vi "ev GoTo.vi"(8 "error in (no error)":errorcluster, 11 "LF2R IDE in":refnum<class "Main Panel.lvclass">) -> (0 "error out":errorcluster, 3 "LF2R IDE out":refnum<class "Main Panel.lvclass">)   [LabVIEW 2018, in "Main Panel.lvlib" / "Main Panel.lvclass"]
uses:
  Main Panel.lvclass
  Main Panel.lvclass/Main Panel.ctl
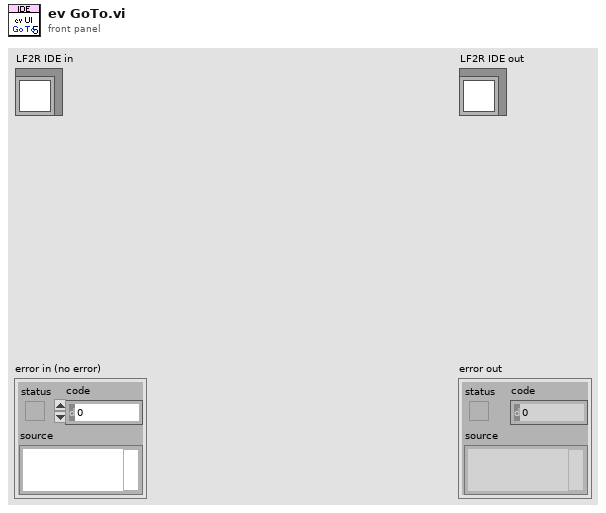
[diagram p1: front panel]
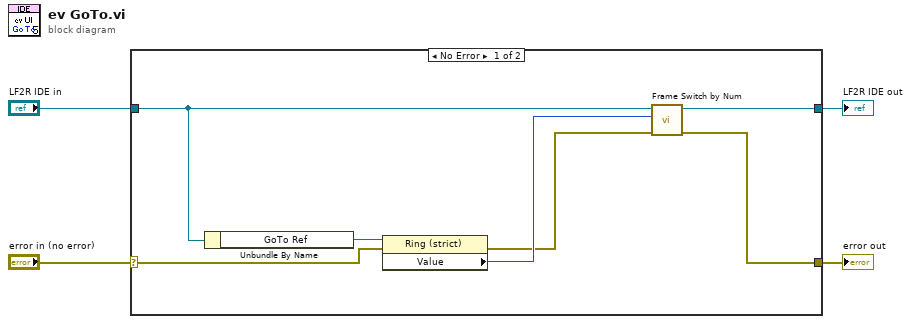
[diagram p0: block diagram]
diagram:
  n1 = case shown="No Error" "error in (no error)" {
    selector: "error in (no error)" -> [w7 w13]
    tunnel: [w5 w13] -> w3
    tunnel: [w6 w12] -> w1
    tunnel: "LF2R IDE in" -> [w10 w12]
    frame No Error {
      n2 = Unbundle By Name(w10) -> ("GoTo Ref"=w11:refnum<vi>)
      n3 = property class="Ring (strict)"(reference=w11, error in=w7) -> (error out=w8:errorcluster, "Value"=w9:u16)  [unwired: 1 out]
      n4 = call "Frame Switch by Num.vi"("error in (no error)"=w8, "Frame Num"=w9, "LF2R IDE in"=w10) -> ("error out"=w5:errorcluster, "LF2R IDE out"=w6:refnum<class "Main Panel.lvclass">)  [unwired: 7 in]
    }
    frame Error {
    }
  }
  "error out" <- w3
  "LF2R IDE out" <- w1
